vi "Auto Start Tasks.vi"(8 "error in":errorcluster) -> (0 "error out":errorcluster, 3 "All Input Tasks":T1)   [LabVIEW 2017]
doc: "Task 1: 1839_AI\n\nTask 2: 1839_DI_1\n\nTask 3: 1839_DI_2"
uses:
  GV/All Inputs.vi
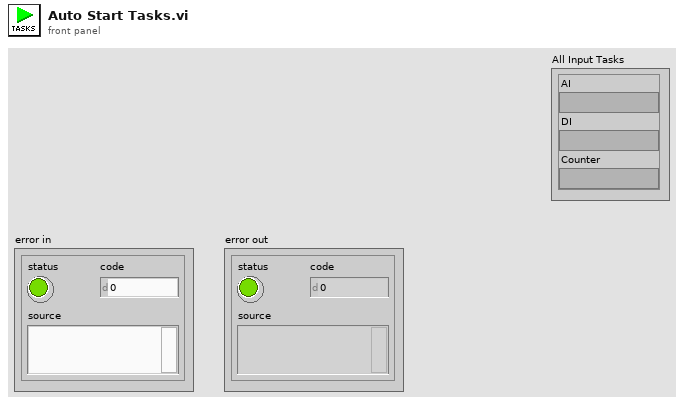
[diagram p1: front panel]
types:
  T1 = cluster{"AI":refnum<k21>, "DI":refnum<k21>, "Counter":refnum<k21>}
  T2 = cluster{"task out":refnum<k21>, "task out":refnum<k21>, "task out":refnum<k21>}
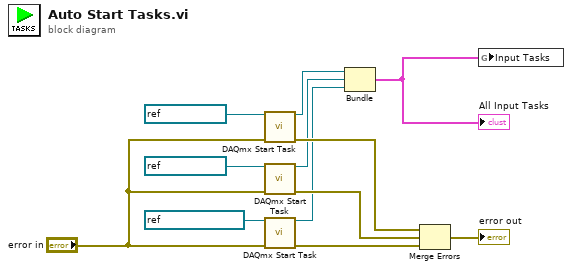
[diagram p0: block diagram]
diagram:
  n1 = call <vilib>:"DAQmx Start Task.vi"("task/channels in"=refnum<k21> "1922_AllAI" ("AI out"), "error in"="error in") -> ("task out"=w4:refnum<k21>, "error out"=w10:errorcluster)  [unwired: 12 in]
  n2 = call <vilib>:"DAQmx Start Task.vi"("task/channels in"=refnum<k21> "1922_AllDI", "error in"="error in") -> ("task out"=w3:refnum<k21>, "error out"=w7:errorcluster)  [unwired: 12 in]
  n3 = call <vilib>:"DAQmx Start Task.vi"("task/channels in"=refnum<k21> "1922_Counter", "error in"="error in") -> ("task out"=w2:refnum<k21>, "error out"=w8:errorcluster)  [unwired: 12 in]
  n4 = Bundle("task out"=w4, "task out"=w3, "task out"=w2) -> (w1:T2)  [unwired: 1 in]
  "All Input Tasks" <- w1
  n5 = Merge Errors(w10, w7, w8) -> (→"error out":errorcluster)
  n6 = global write "All Inputs.vi" "Input Tasks"(w1) -> ()
